vi "rad_Format Target Information.vi"(11 "Targets Information":T1[](array[typedef]) {"Primary NIC"."IP Address Request Mode" items=["Static"=1, "DHCP/Link-Local"=2, "Link-Local Only"=4, "DHCP Only"=8]}) -> (3 "Targets Information":string[][](array[string]))   [LabVIEW 2016]
uses:
  TypeDefs/rad_Target Information.ctl
  TypeDefs/rad_Target Network Settings.ctl
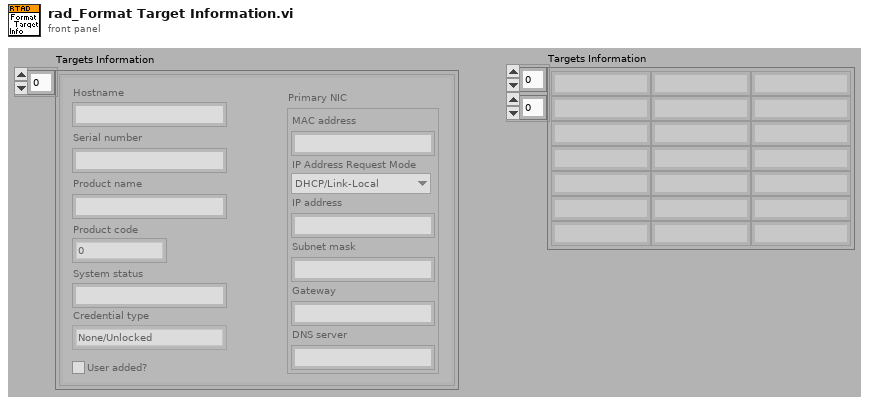
[diagram p1: front panel]
types:
  T1 = typedef "rad_Target Information.ctl" = cluster{"Hostname":string, "Serial number":string, "Product name":string, "Product code":i32, "System status":string, "Credential type":enum16{"None/Unlocked", "FTP Password", "NIAuth Credentials"}, "User added?":bool, "Primary NIC":T2}
  T2 = typedef "rad_Target Network Settings.ctl" = cluster{"MAC address":string, "IP Address Request Mode":i32, "IP address":string, "Subnet mask":string, "Gateway":string, "DNS server":string}
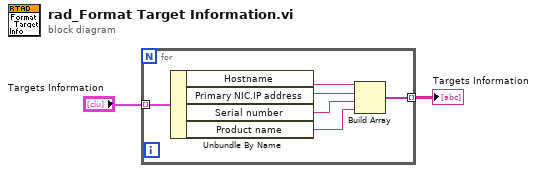
[diagram p0: block diagram]
diagram:
  n1 = for {
    tunnel: "Targets Information" -> [w8] mode=indexing
    tunnel: [w4] -> w2 mode=indexing
    n2 = Unbundle By Name(w8) -> ("Hostname"=w7:string, "Primary NIC.IP address"=w6:string, "Serial number"=w3:string, "Product name"=w5:string)
    n3 = Build Array(w7, w6, w3, w5) -> (w4:string[])
  }
  "Targets Information" <- w2
